vi "DAQ_Manager.GetEvents.vi"(8 "error in (no error)":errorcluster, 11 "DAQ_Manager in":refnum<class "DAQ_Manager.lvclass">) -> (0 "error out":errorcluster, 3 "DAQ_Manager":cluster{"Public Events":T1, "Public Events":T2})   [LabVIEW 2016, in "DAQ_Manager.lvclass"]
uses:
  DAQ_Manager.lvclass
  <vilib>/JKI/JKI SMO/SMO/Typedefs/Public Events.ctl
  <vilib>/JKI/JKI SMO/SMO/Typedefs/SMOState --Enum.ctl
  <vilib>/JKI/JKI SMO/SMO/Typedefs/Reserve State--Enum.ctl
  Typedefs/PublicEvents--Cluster.ctl
  Typedefs/PublicEvents--DAQ_Manager.getWaveform.ctl
  C:/Program Files (x86)/National Instruments/LabVIEW 2016/vi.lib/JKI/JKI SMO/SMO/SMO.lvclass
  <vilib>/JKI/JKI SMO/SMO/SMO.lvclass
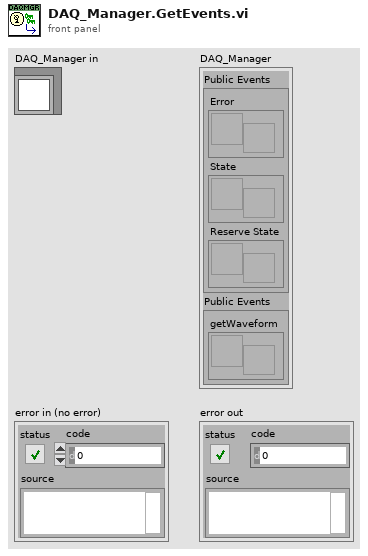
[diagram p1: front panel]
types:
  T1 = typedef "SMO.lvclass/Public Events.ctl" = cluster{"Error":refnum<user-event>, "State":refnum<user-event>, "Reserve State":refnum<user-event>}
  T2 = typedef "DAQ_Manager.lvclass/PublicEvents--Cluster.ctl" = cluster{"getWaveform":refnum<user-event>}
  T3 = cluster{"Public Events":T1, "DAQManager.Public Events":T2}
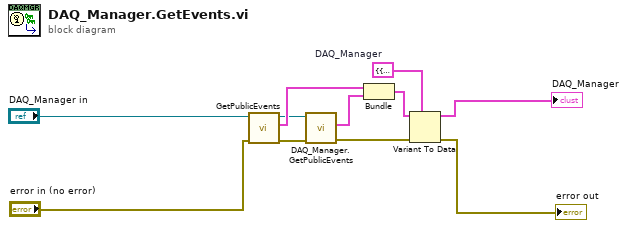
[diagram p0: block diagram]
diagram:
  w8 = cluster{"Public Events":T1, "Public Events":T2} {"Public Events"={"Error"=refnum, "State"=refnum, "Reserve State"=refnum}, "Public Events"={"getWaveform"=refnum}}  # DAQ_Manager
  n1 = call <vilib>:"GetPublicEvents.vi"("error in (no error)"="error in (no error)", "SMO"="DAQ_Manager in") -> ("error out"=w6:errorcluster, "Public Events"=w4:T1, "SMO out"=w3:refnum<class "DAQ_Manager.lvclass">)  [unwired: 7 in]
  n2 = call "DAQ_Manager.GetPublicEvents.vi"("error in (no error)"=w6, "DAQ_Manager"=w3) -> ("error out"=w10:errorcluster, "DAQManager.Public Events"=w5:T2)  [unwired: 7 in, 1 out]
  n3 = Bundle("Public Events"=w4, "DAQManager.Public Events"=w5) -> (w7:T3)  [unwired: 1 in]
  n4 = Variant To Data(error in=w10, type=w8, Variant=w7) -> (data=→"DAQ_Manager":cluster{"Public Events":T1, "Public Events":T2}, error out=→"error out":errorcluster)
